vi "Main-数据保存.vi"(5 "ModelEditInfo":T2={"AllModelFold"=path "", "AllModelNamePath"=path "", "所有零件型号"=[], "当前零件型号"="", "所有建立零件信息"=[], "当前零件序号"=0, "当前产品信息"={"产品型号"="J016-9STWH-A插头", "二维码拍照"=0, "Mark点拍照"=0}}, 6 "错误常量in":errorcluster caption="错误常量", 7 "存档数据和结果":T1, 9 "选项":T4) -> (0 "错误常量out":errorcluster caption="错误常量")   [LabVIEW 2014]
uses:
  SaveTestDataAction.ctl
  ModelEditSubVIs/ModeEditeControl.ctl
  ModelEditSubVIs/ModelInfo.ctl
  Controls/MsgAction.ctl
  Global.vi
panel:
  out "当天存数据路径":path
  out "time":u32
  out "添加的路径":path
  out "数据存储路径":path
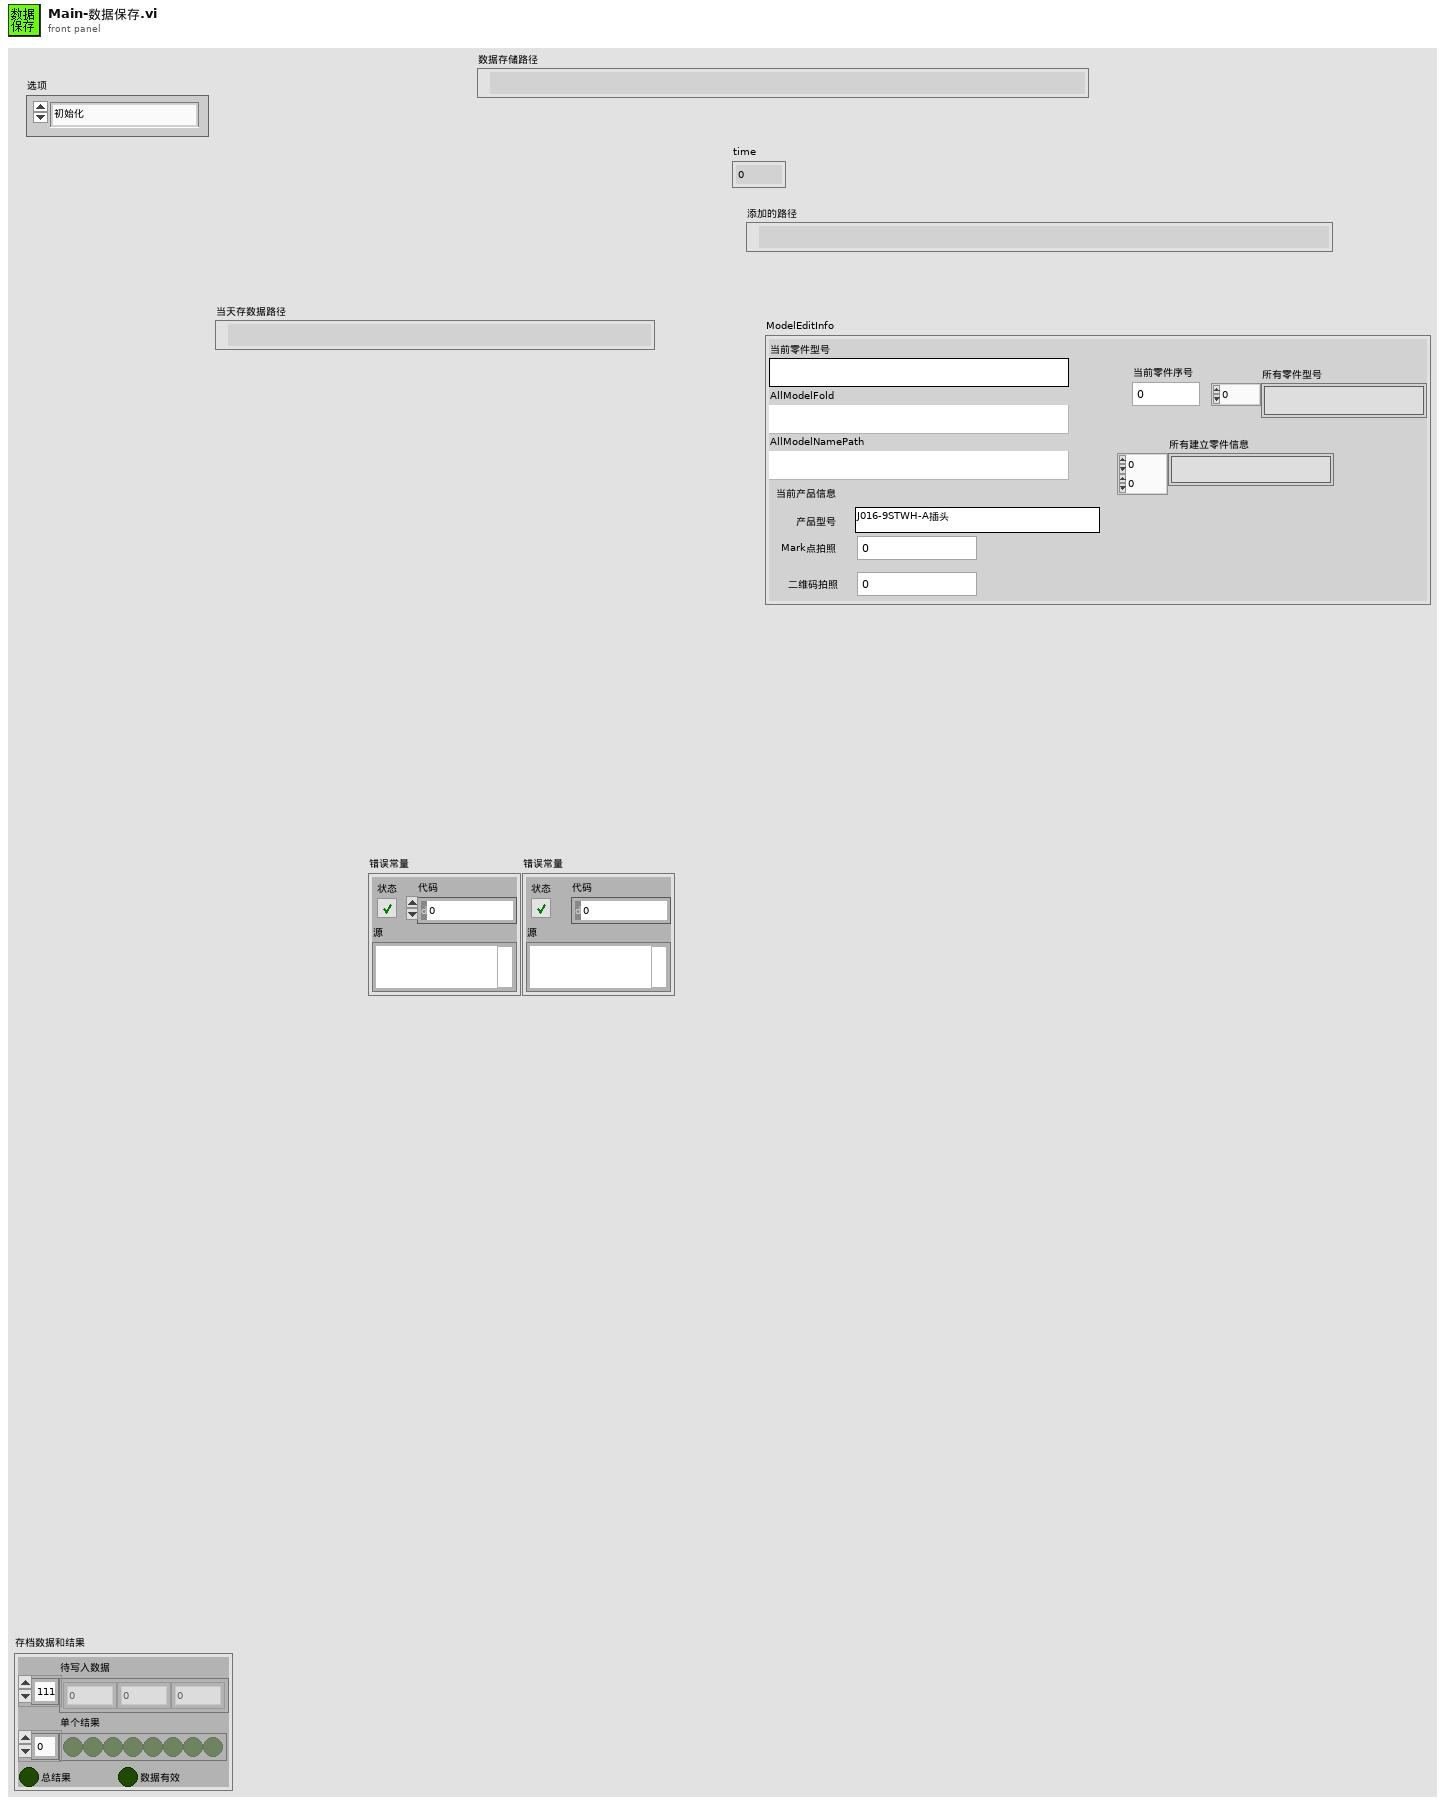
[diagram p1: front panel]
types:
  T1 = typedef "存档数据和结果.ctl" = cluster{"待写入数据":dbl[], "单个结果":bool[], "总结果":bool, "数据有效":bool}
  T2 = typedef "ModeEditeControl.ctl" = cluster{"AllModelFold":path, "AllModelNamePath":path, "所有零件型号":string[], "当前零件型号":string, "所有建立零件信息":string[][], "当前零件序号":i32, "当前产品信息":T3}
  T3 = typedef "ModelInfo.ctl" = cluster{"产品型号":string, "二维码拍照":u32, "Mark点拍照":u32}
  T4 = typedef "SaveTestDataAction.ctl" = enum16{"初始化", "更新机种规格", "读取表格", "第N次拍照数据写入表格(缓存)", "Mark点拍照数据存档", "取料拍螺帽数据存档", "复锁拍螺帽数据存档", "关闭表格", "打开表格"}
  T5 = typedef "OtherSpec.ctl" = cluster{"其它勾选类规格":T6, "其它数据类规格":T7, "相机名称":T8, "参数":cluster{"Mark1曝光时间":i32, "Mark2曝光时间":i32, "二维码曝光时间":i32}}
  T6 = typedef "其它勾选类规格.ctl" = cluster{"保存图片":bool, "上传设备状态数据":bool, "保存数据":bool, "开机默认开启监控摄像头":bool, "启用mark拍照 ":bool}
  T7 = typedef "其他数据类规格.ctl" = cluster{"相机1像素-毫米换算系数":dbl, "相机2像素-毫米换算系数":dbl, "D盘剩余空间预警(G)":dbl, "视频最长录制时间(秒)":dbl}
  T8 = typedef "相机名称品牌使用状态.ctl" = cluster{"相机1名称":T9, "相机2名称":T9, "Cam1启用":bool, "Cam2启用":bool, "Basler1":bool, "Basler2":bool}
  T9 = typedef "IMAQdx.ctl" = refnum<k21>
  T10 = typedef "MsgAction.ctl" = enum16{"初始化", "添加消息", "区分结果添加消息", "清空消息", "获取消息"}
  T11 = typedef "控件-Excel读写选项.ctl" = enum16{"打开表格", "新增sheet", "读取sheet指定位置数据", "读取sheet整个数据", "写入sheet整个数据", "写表头", "数据存到本机", "表格是否开启状态", "关闭表格"}
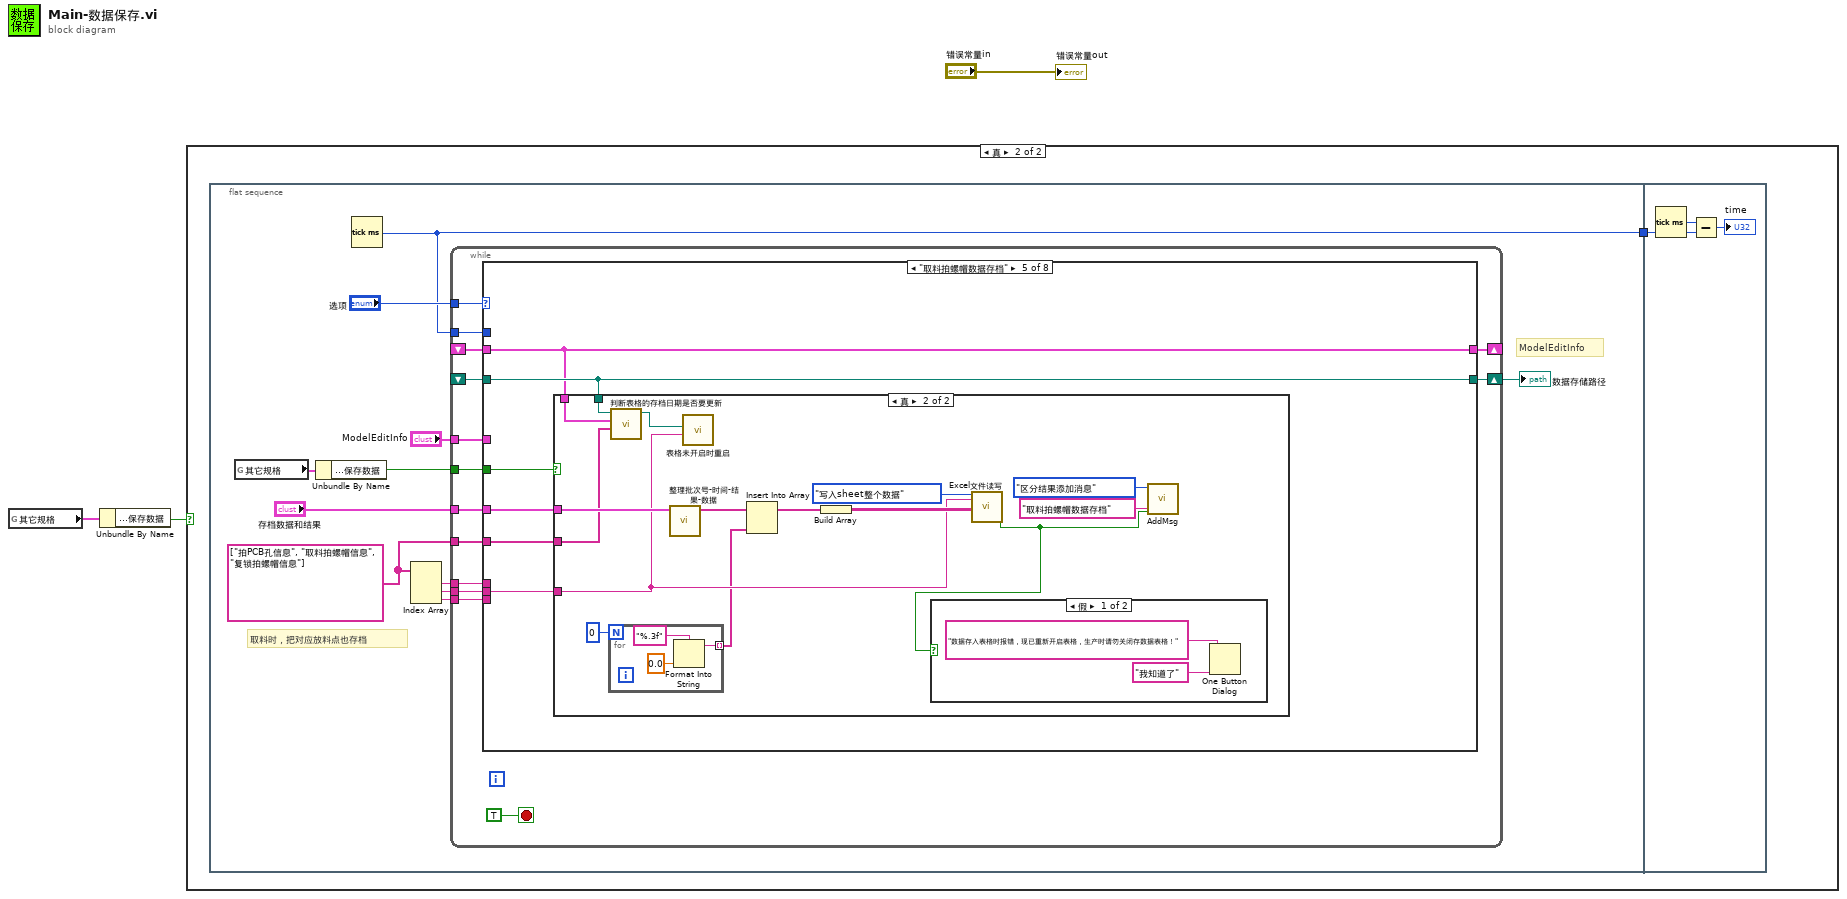
[diagram p0: block diagram]
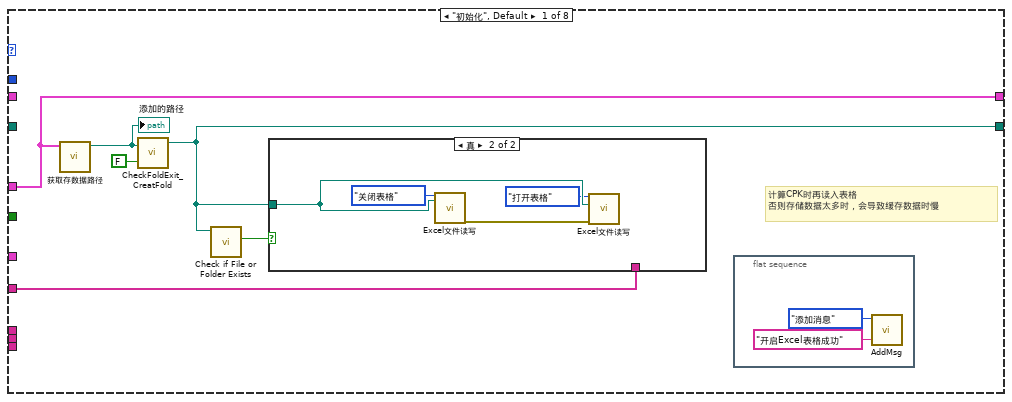
[diagram p3: hidden frame]
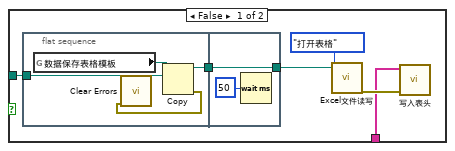
[diagram p4: hidden frame]
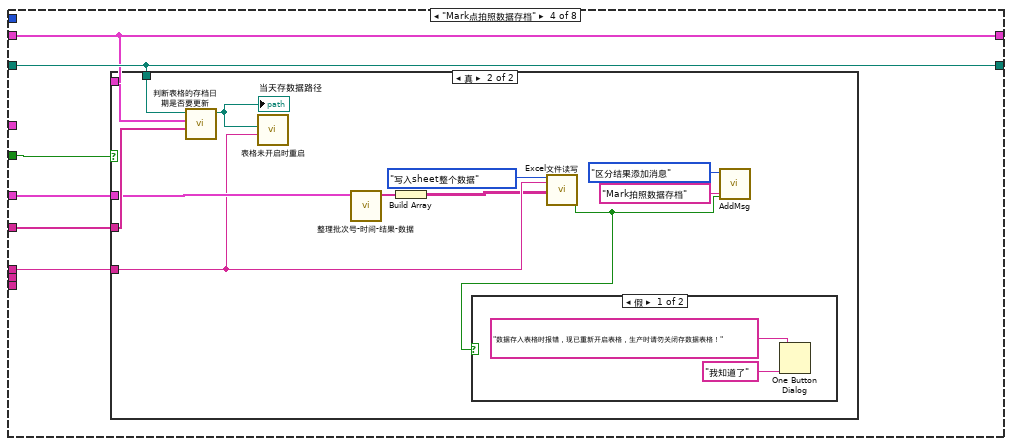
[diagram p7: hidden frame]
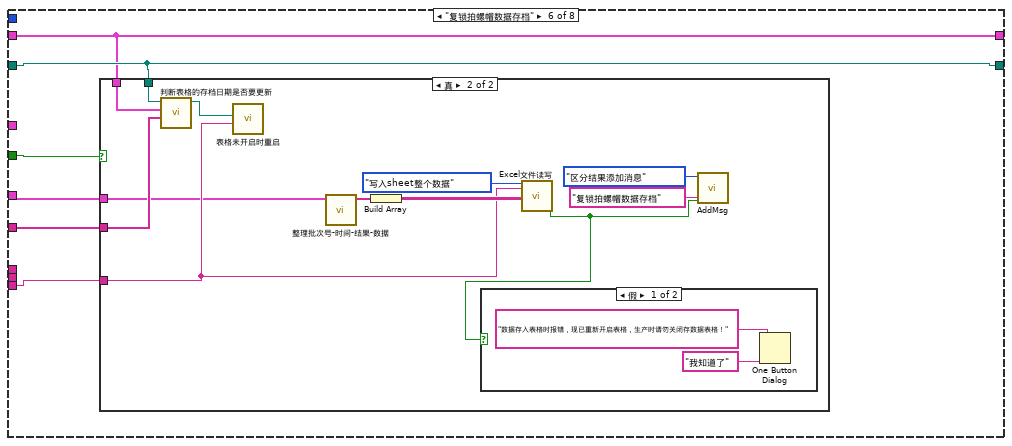
[diagram p12: hidden frame]
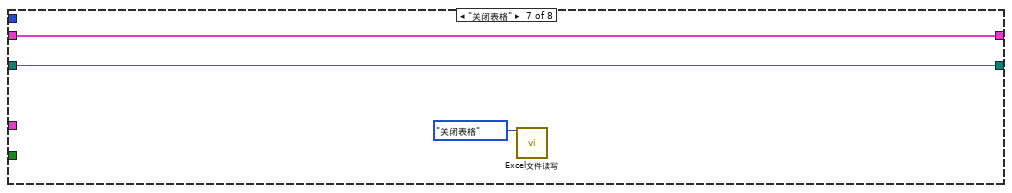
[diagram p15: hidden frame]
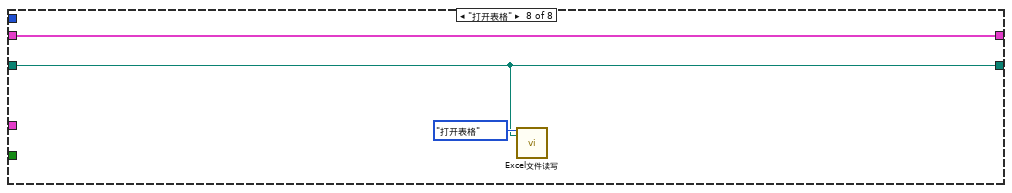
[diagram p16: hidden frame]
diagram:
  n1 = global read "Global.vi" "其它规格"() -> (w2:T5)
  n2 = Unbundle By Name(w2) -> ("其它勾选类规格.保存数据"=w1:bool)
  n3 = case shown="真" w1 {
    frame False {
    }
    frame True {
      n4 = flat-sequence {
        tunnel: [w10] -> w4
        tunnel: w4 -> [w131]
        frame #0 {
          w9 = string[] ["拍PCB孔信息", "取料拍螺帽信息", "复锁拍螺帽信息"]
          # "取料时，把对应放料点也存档"
          # "ModelEditInfo"
          n5 = global read "Global.vi" "其它规格"() -> (w6:T5)
          n6 = Unbundle By Name(w6) -> ("其它勾选类规格.保存数据"=w5:bool)
          n7 = Tick Count (ms)() -> (millisecond timer value=w10:u32)
          n8 = Index Array(array=w9) -> (element #1=w12:string, element #2=w8:string, element #3=w7:string)  [unwired: 3 in]
          n9 = while {
            tunnel: "选项" -> [w28]
            shift-right: [w27] -> w14
            shift-left: _ -> [w26]
            tunnel: "ModelEditInfo" -> [w25]
            tunnel: w9 -> [w24]
            shift-right: [w23] -> _
            shift-left: _ -> [w22]
            tunnel: w12 -> [w21]
            tunnel: "存档数据和结果" -> [w20]
            tunnel: w10 -> [w19]
            tunnel: w8 -> [w18]
            tunnel: w7 -> [w17]
            tunnel: w5 -> [w16]
            stop <- TRUE stop-if-true
            n10 = case shown="\"取料拍螺帽数据存档\"" w28 {
              tunnel: [w35 w54 w56 w63 w82 w108 w126 w127] -> w27
              tunnel: w26 -> [_ w54 w56 w63 w82 w108 w126 w127]
              tunnel: w25 -> [w30 w55 _ _ _ _ _ _]
              tunnel: w24 -> [w34 _ _ w61 w80 w106 _ _]
              tunnel: [w30 w55 w57 w62 w81 w107 w125 w129] -> w23
              tunnel: w22 -> [_ _ w57 w62 w81 w107 w125 w129]
              tunnel: w21 -> [_ _ _ w59 _ _ _ _]
              tunnel: w20 -> [_ _ _ w60 w83 w105 _ _]
              tunnel: w19 -> [_ _ _ _ _ _ _ _]
              tunnel: w18 -> [_ _ _ _ w79 _ _ _]
              tunnel: w17 -> [_ _ _ _ _ w109 _ _]
              tunnel: w16 -> [_ _ _ w58 w78 w104 _ _]
              frame "初始化", Default {
                # "计算CPK时再读入表格\n否则存储数据太多时，会导致缓存数据时慢"
                n11 = call "获取存数据路径.vi"("ModelEditInfo"=w30) -> ("当天存数据路径"=w32:path)  [unwired: 10 in]
                "添加的路径" <- w32
                n12 = call "CheckFoldExit_CreatFold.vi"("path in"=w32, "FoldOrFile¡H"=FALSE) -> ("File out"=w35:path)  [unwired: 2 out]
                n13 = call <vilib>:"Check if File or Folder Exists.vi"("path"=w35) -> ("file or folder exists?"=w31:bool)  [unwired: 1 in, 9 out]
                n14 = case shown="真" w31 {
                  tunnel: w35 -> [w42 w52]
                  tunnel: w34 -> [w38 _]
                  frame False {
                    n15 = flat-sequence {
                      tunnel: w42 -> [w47]
                      tunnel: [w45] -> w43
                      tunnel: w43 -> [w48]
                      tunnel: [w48] -> w41
                      frame #0 {
                        n16 = global read "Global.vi" "数据保存表格模板"() -> (w46:path)
                        n17 = Copy(10:w47, 11:w46) -> (0:w44:errorcluster, 3:w45:path)  [unwired: 3 in, 1 out]
                        n18 = call <vilib>:"Clear Errors.vi"("error in (no error)"=w44) -> ()  [unwired: 5 in, 2 out]
                      }
                      frame #1 {
                        n19 = Wait (ms)(milliseconds to wait=u32 50 ("等待时间（毫秒）")) -> ()  [unwired: 1 out]
                      }
                    }
                    n20 = call "Excel文件读写.vi"("选项"=控件-Excel读写选项."打开表格", "Path"=w41) -> ("error out"=w39:errorcluster)  [unwired: 15 in, 2 out]
                    n21 = call "写入表头.vi"("错误in"=w39, "各sheet名称数组"=w38) -> ()  [unwired: 10 in]
                  }
                  frame True {
                    n22 = call "Excel文件读写.vi"("选项"=控件-Excel读写选项."关闭表格", "Path"=w52) -> ("error out"=w53:errorcluster)  [unwired: 15 in, 2 out]
                    n23 = call "Excel文件读写.vi"("选项"=控件-Excel读写选项."打开表格", "error in"=w53, "Path"=w52) -> ()  [unwired: 14 in, 3 out]
                  }
                }
                n24 = flat-sequence {
                  frame #0 {
                    n25 = call "AddMsg.vi"("添加消息"="开启Excel表格成功", "消息Action"=MsgAction."添加消息") -> ()  [unwired: 2 in, 1 out]
                  }
                }
              }
              frame "更新机种规格" {
              }
              frame "读取表格" {
              }
              frame "Mark点拍照数据存档" {
                n26 = case shown="真" w58 {
                  tunnel: w63 -> [_ w74]
                  tunnel: w62 -> [_ w73]
                  tunnel: w61 -> [_ w72]
                  tunnel: w60 -> [_ w71]
                  tunnel: w59 -> [_ w70]
                  frame False {
                  }
                  frame True {
                    n27 = call "判断表格的存档日期是否要更新.vi"("各Sheet名称数组"=w72, "ModelEditInfo输入"=w73, "已经存在路径"=w74) -> ("当天存数据路径"=w75:path)  [unwired: 7 in, 1 out]
                    "当天存数据路径" <- w75
                    n28 = call "表格未开启时重启.vi"("worksheet name"=w70, "Path"=w75) -> ()  [unwired: 8 in, 2 out]
                    n29 = call "整理批次号-时间-结果-数据.vi"("存档数据和结果"=w71) -> ("数组"=w68:string[])  [unwired: 9 in, 1 out]
                    n30 = Build Array(w68) -> (w67:string[][])
                    n31 = call "Excel文件读写.vi"("选项"=控件-Excel读写选项."写入sheet整个数据", "sheet name"=w70, "表格"=w67) -> ("表格操作正常"=w64:bool)  [unwired: 14 in, 2 out]
                    n32 = case shown="假" w64 {
                      frame False {
                        n33 = One Button Dialog(message="数据存入表格时报错，现已重新开启表格，生产时请勿关闭存数据表格！" ("消息"), button name ("OK")="我知道了" ("按钮名称（“确定”）")) -> ()  [unwired: 1 out]
                      }
                      frame True {
                      }
                    }
                    n34 = call "AddMsg.vi"("Result"=w64, "添加消息"="Mark拍照数据存档", "消息Action"=MsgAction."区分结果添加消息") -> ()  [unwired: 1 in, 1 out]
                  }
                }
              }
              frame "取料拍螺帽数据存档" {
                n35 = case shown="真" w78 {
                  tunnel: w83 -> [_ w92]
                  tunnel: w82 -> [_ w91]
                  tunnel: w81 -> [_ w90]
                  tunnel: w80 -> [_ w89]
                  tunnel: w79 -> [_ w88]
                  frame False {
                  }
                  frame True {
                    n36 = for {
                      N: 0 -> [_]
                      tunnel: [w101] -> w85 mode=indexing
                      n37 = Format Into String(format string="%.3f" ("格式字符串"), 0.0 ("输入 1")) -> (resulting string=w101:string)  [unwired: 2 in, 1 out]
                    }
                    n38 = call "判断表格的存档日期是否要更新.vi"("各Sheet名称数组"=w89, "ModelEditInfo输入"=w90, "已经存在路径"=w91) -> ("当天存数据路径"=w98:path)  [unwired: 7 in, 1 out]
                    n39 = call "整理批次号-时间-结果-数据.vi"("存档数据和结果"=w92) -> ("数组"=w87:string[])  [unwired: 9 in, 1 out]
                    n40 = call "表格未开启时重启.vi"("worksheet name"=w88, "Path"=w98) -> ()  [unwired: 8 in, 2 out]
                    n41 = Insert Into Array(array=w87, new element=w85) -> (w86:string[])  [unwired: 1 in]
                    n42 = Build Array(w86) -> (w96:string[][])
                    n43 = call "Excel文件读写.vi"("选项"=控件-Excel读写选项."写入sheet整个数据", "sheet name"=w88, "表格"=w96) -> ("表格操作正常"=w93:bool)  [unwired: 14 in, 2 out]
                    n44 = case shown="假" w93 {
                      frame False {
                        n45 = One Button Dialog(message="数据存入表格时报错，现已重新开启表格，生产时请勿关闭存数据表格！" ("消息"), button name ("OK")="我知道了" ("按钮名称（“确定”）")) -> ()  [unwired: 1 out]
                      }
                      frame True {
                      }
                    }
                    n46 = call "AddMsg.vi"("Result"=w93, "添加消息"="取料拍螺帽数据存档", "消息Action"=MsgAction."区分结果添加消息") -> ()  [unwired: 1 in, 1 out]
                  }
                }
              }
              frame "复锁拍螺帽数据存档" {
                n47 = case shown="真" w104 {
                  tunnel: w109 -> [_ w114]
                  tunnel: w108 -> [_ w113]
                  tunnel: w107 -> [_ w112]
                  tunnel: w106 -> [_ w111]
                  tunnel: w105 -> [_ w110]
                  frame False {
                  }
                  frame True {
                    n48 = call "判断表格的存档日期是否要更新.vi"("各Sheet名称数组"=w111, "ModelEditInfo输入"=w112, "已经存在路径"=w113) -> ("当天存数据路径"=w121:path)  [unwired: 7 in, 1 out]
                    n49 = call "表格未开启时重启.vi"("worksheet name"=w114, "Path"=w121) -> ()  [unwired: 8 in, 2 out]
                    n50 = call "整理批次号-时间-结果-数据.vi"("存档数据和结果"=w110) -> ("数组"=w119:string[])  [unwired: 9 in, 1 out]
                    n51 = Build Array(w119) -> (w118:string[][])
                    n52 = call "Excel文件读写.vi"("选项"=控件-Excel读写选项."写入sheet整个数据", "sheet name"=w114, "表格"=w118) -> ("表格操作正常"=w115:bool)  [unwired: 14 in, 2 out]
                    n53 = case shown="假" w115 {
                      frame False {
                        n54 = One Button Dialog(message="数据存入表格时报错，现已重新开启表格，生产时请勿关闭存数据表格！" ("消息"), button name ("OK")="我知道了" ("按钮名称（“确定”）")) -> ()  [unwired: 1 out]
                      }
                      frame True {
                      }
                    }
                    n55 = call "AddMsg.vi"("Result"=w115, "添加消息"="复锁拍螺帽数据存档", "消息Action"=MsgAction."区分结果添加消息") -> ()  [unwired: 1 in, 1 out]
                  }
                }
              }
              frame "关闭表格" {
                n56 = call "Excel文件读写.vi"("选项"=控件-Excel读写选项."关闭表格") -> ()  [unwired: 16 in, 3 out]
              }
              frame "打开表格" {
                n57 = call "Excel文件读写.vi"("选项"=控件-Excel读写选项."打开表格", "Path"=w127) -> ()  [unwired: 15 in, 3 out]
              }
            }
          }
          "数据存储路径" <- w14
        }
        frame #1 {
          n58 = Tick Count (ms)() -> (millisecond timer value=w132:u32)
          n59 = Subtract(x=w132, y=w131) -> (x-y=→"time":u32)
        }
      }
    }
  }
  "错误常量out" <- "错误常量in"
